vi "PAT Device Software 1.3.vi"() -> ()   [LabVIEW 2018]
uses:
  <vilib>/Utility/error.llb/DialogType.ctl
  <vilib>/DAQmx/write.llb/DAQmx Write (Analog 1D DBL NChan 1Samp).vi
  <vilib>/DAQmx/read.llb/DAQmx Read (Analog 1D DBL NChan 1Samp).vi
  <vilib>/DAQmx/write.llb/DAQmx Write (Analog DBL 1Chan 1Samp).vi
  <vilib>/Analysis/baseanly.llb/Mean (DBL).vi
  <vilib>/Instr/_visa.llb/VISA Configure Serial Port (Instr).vi
  <vilib>/DAQmx/create/channels.llb/DAQmx Create Channel (AO-Voltage-Basic).vi
  <vilib>/DAQmx/create/channels.llb/DAQmx Create Channel (AI-Voltage-Basic).vi
  <vilib>/DAQmx/configure/timing.llb/DAQmx Timing (Sample Clock).vi
  <vilib>/DAQmx/miscellaneous.llb/DAQmx Fill In Error Info.vi
  <vilib>/Analysis/NI_AALBase.lvlib
panel:
  out "CV2 Voltage":dbl format="%#_13g"
  out "CV1 Voltage":dbl format="%#_13g"
  in  "In Progress":bool
  out "Total Test Time":i32
  in  "Test Buffer Duration":i32=10
  in  "Motor Control":bool
  out "Corrected Voltage":dbl=3.0 format="%#_13g"
  out "Rotation Time":dbl format="%#_3g"
  out "Error Ratio":dbl format="%#_13g"
  out "Reference Voltage":dbl=3.001413381851861 format="%0.2f"
  in  "Target Rotation Time":dbl=2.8 format="%#_13g"
  out "Hit Recorded":bool
  in  "CV2 Output":tag="Dev1/ao0"
  in  "CV1 Output":tag="Dev1/ao1"
  in  "Motor Output":tag="Dev2/ao0"
  in  "Hall Sensor Channel":tag="Dev2/ai3"
  in  "O2 Channel":tag="Dev2/ai2"
  in  "P2 Channel":tag="Dev2/ai1"
  in  "PA Channel":tag="Dev2/ai0"
  in  "Relay Port":refnum<visa-resource-name>="COM9"
  in  "Reset To Default":bool
  in  "Sample Rate":i32=10
  in  "CV2 Channel":tag="Dev1/ai0"
  in  "CV1 Channel":tag="Dev1/ai1"
  in  "TA Channel":tag="Dev1/ai6"
  in  "RHA Channel":tag="Dev1/ai7"
  in  "P1 Channel":tag="Dev1/ai5"
  out "Stop Test":bool=TRUE
  out "Is PAT Test?":bool
  in  "Test Begin":bool
  out "Test Duration":i32
  out "Current Test":string
  out "Test Underway":i32
  out "Number of tests":i32=4
  out "Test List":i16[](array[numeric])=[1, 1, 1, 1, 0, 0]
  out "error out 3":errorcluster
  in  "error in 2":errorcluster
  out "error out 2":errorcluster
  in  "error in":errorcluster
  out "error out":errorcluster
  in  "error in (no error)":errorcluster
  in  "Tab Control":enum32{"PAT Test", "Manual Control"}(tab)
  out "PAT Test Readings":T1 {"B40 S" scale=0.0..100.0; "B15 S" scale=0.0..100.0; "Ex70 S" scale=0.0..100.0; "Ex30 S" scale=0.0..100.0; "In70 S" scale=0.0..100.0; "In30 S" scale=0.0..100.0}
  out "Status":string="Status"
  out "Time":string="Time (s)"
  out "Limit":string="Limit"
  out "Comp":string="Comp"
  out "Units":string="Units"
  out "Measured":string="Measured"
  out "Test Name":string="Test Name"
  out "String 22":string="-0.8"
  out "String 24":string="0.8"
  out "String 23":string="-2.0"
  out "String 26":string="26"
  out "String 25":string="2.0"
  out "String 27":string="89"
  out "String 15":string=">="
  out "String 17":string="<="
  out "String 16":string=">="
  out "String 19":string=">="
  out "String 18":string="<="
  out "String 20":string=">="
  out "String 8":string="in H2O"
  out "String 10":string="in H2O"
  out "String 9":string="in H2O"
  out "String 12":string="% O2"
  out "String 11":string="in H2O"
  out "String 13":string="% O2"
  out "String":string="Inhalation (30lpm)"
  out "String 3":string="Exhalation (30lpm)"
  out "String 2":string="Inhalation (70lpm)"
  out "String 5":string="Breathing (15kft)"
  out "String 4":string="Exhalation (70lpm)"
  out "String 6":string="Breathing (40kft)"
  in  "Start PAT Test":bool
  in  "Stop PAT Test":bool
  out "Test Status:":string
  in  "Results File Location:":path=path "X:/Working/Finn Sowerbutts/Aerox/PAT/CDR Files/PAT Device Software/Test Reports"
  in  "PAT Test Settings":T2={"Test Date:"="24 Jan 2019", "Test Time:"="11:23:54", "Pull Test Date:"="", "Operator:"="", "Production Order No.:"="", "Production Lot:"="", "No. Masks in Lot:"="", "Comments:"="", "Array"=[TRUE, TRUE, TRUE, TRUE, FALSE, FALSE], "Test Parameters:"=enum."Quick Test", "Facepiece Leakage"=0.0}
  in  "Preset Directory:":path=path "X:/Working/Finn Sowerbutts/Aerox/PAT/CDR Files/PAT Device Software/Presets"
  in  "MC Fields":T3={"Test Date:"="24 Jan 2019", "Test Time:"="11:23:54", "Operator:"="", "PAX Serial No.:"="", "Production Lot:"="", "No. Masks in Lot:"="", "Test Duration"=0, "Presets in Directory:"=0, "MC Test Length"=enum."Run Continuously", "Current Preset:"="Breathing Test 2.ini", "Preset Save"=FALSE}
  in  "MC Instrumentation":T4 {"Motor Speed:" min=0.0 max=3.0 step=0.25; "F2 Leakage" min=0.0 max=150.0 step=1.0; "CV2 Flow Rate:" min=0.0 max=100.0 step=10.0; "CV1 Flow Rate:" min=0.0 max=5.0 step=0.5}
  in  "Start Custom Test":bool
  in  "Stop Custom Test":bool
  # "ccm"
  # "s"
  # "Pamb"
  # "Tamb"
  # "Hamb"
  # "in H2O"
  # "°C"
  # "%"
  # "F2"
  # "ccm"
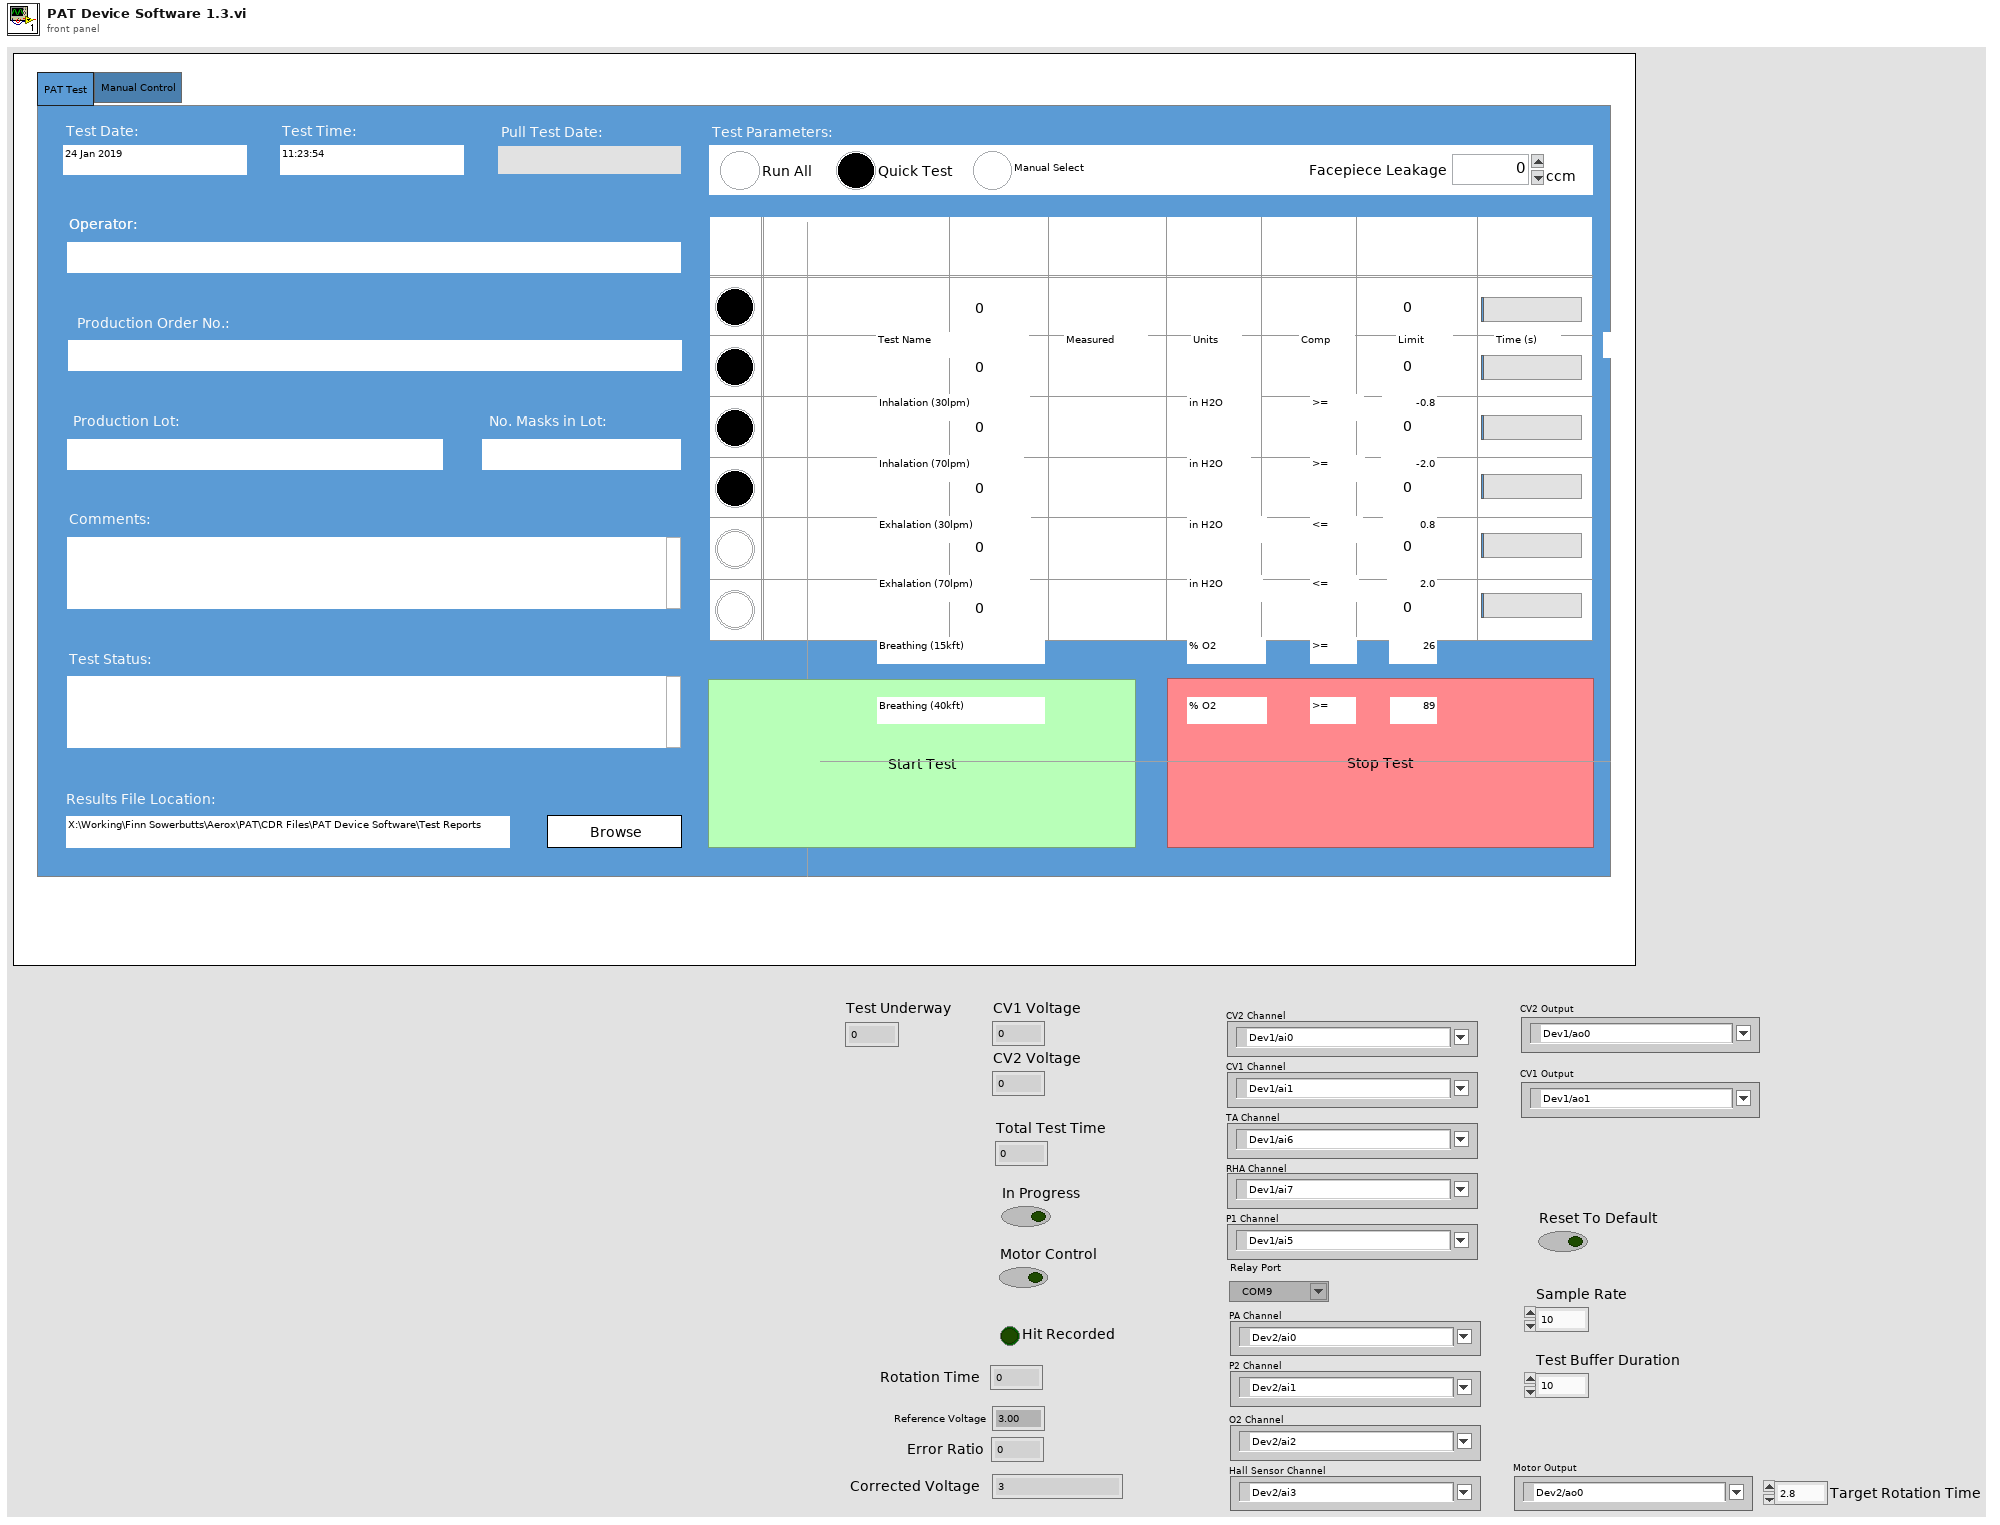
[diagram p1: front panel]
types:
  T1 = cluster{"In30 M":dbl, "In30 T":i64, "In30 S":u8, "In70 M":dbl, "Ex30 M":dbl, "Ex70 M":dbl, "B40 M":dbl, "B15 M":dbl, "In70 T":i64, "Ex30 T":i64, "Ex70 T":i64, "B40 T":i64, "B15 T":i64, "In70 S":u8, "Ex30 S":u8, "Ex70 S":u8, "B15 S":u8, "B40 S":u8}
  T2 = cluster{"Test Date:":string, "Test Time:":string, "Pull Test Date:":string, "Operator:":string, "Production Order No.:":string, "Production Lot:":string, "No. Masks in Lot:":string, "Comments:":string, "Array":bool[], "Test Parameters:":enum32{"Run All", "Quick Test", "Manual Select"}, "Facepiece Leakage":dbl}
  T3 = cluster{"Test Date:":string, "Test Time:":string, "Operator:":string, "PAX Serial No.:":string, "Production Lot:":string, "No. Masks in Lot:":string, "Test Duration":i64, "Presets in Directory:":i32, "MC Test Length":enum32{"Run Continuously", "Run for:"}, "Current Preset:":string, "Preset Save":bool}
  T4 = cluster{"SV1":bool, "SV2":bool, "SV3":bool, "SV4":bool, "SV5":bool, "SV6":bool, "SV7":bool, "SV8":bool, "SV9":bool, "M1":bool, "MP1":bool, "MP2":bool, "CV1":bool, "CV2":bool, "CV1 Flow Rate:":dbl, "CV2 Flow Rate:":dbl, "P2 Pressure:":dbl, "O2 Concentration:":dbl, "Ambient Pressure:":dbl, "Ambient Temp.:":dbl, "Ambient Humidity:":dbl, "Motor Speed:":dbl, "F2 Leakage":dbl, "P1 Pressure:":dbl}
  T5 = enum8{"Enabled", "Disabled", "Disabled and Grayed Out"}
  T6 = typedef "DialogType.ctl" = u16
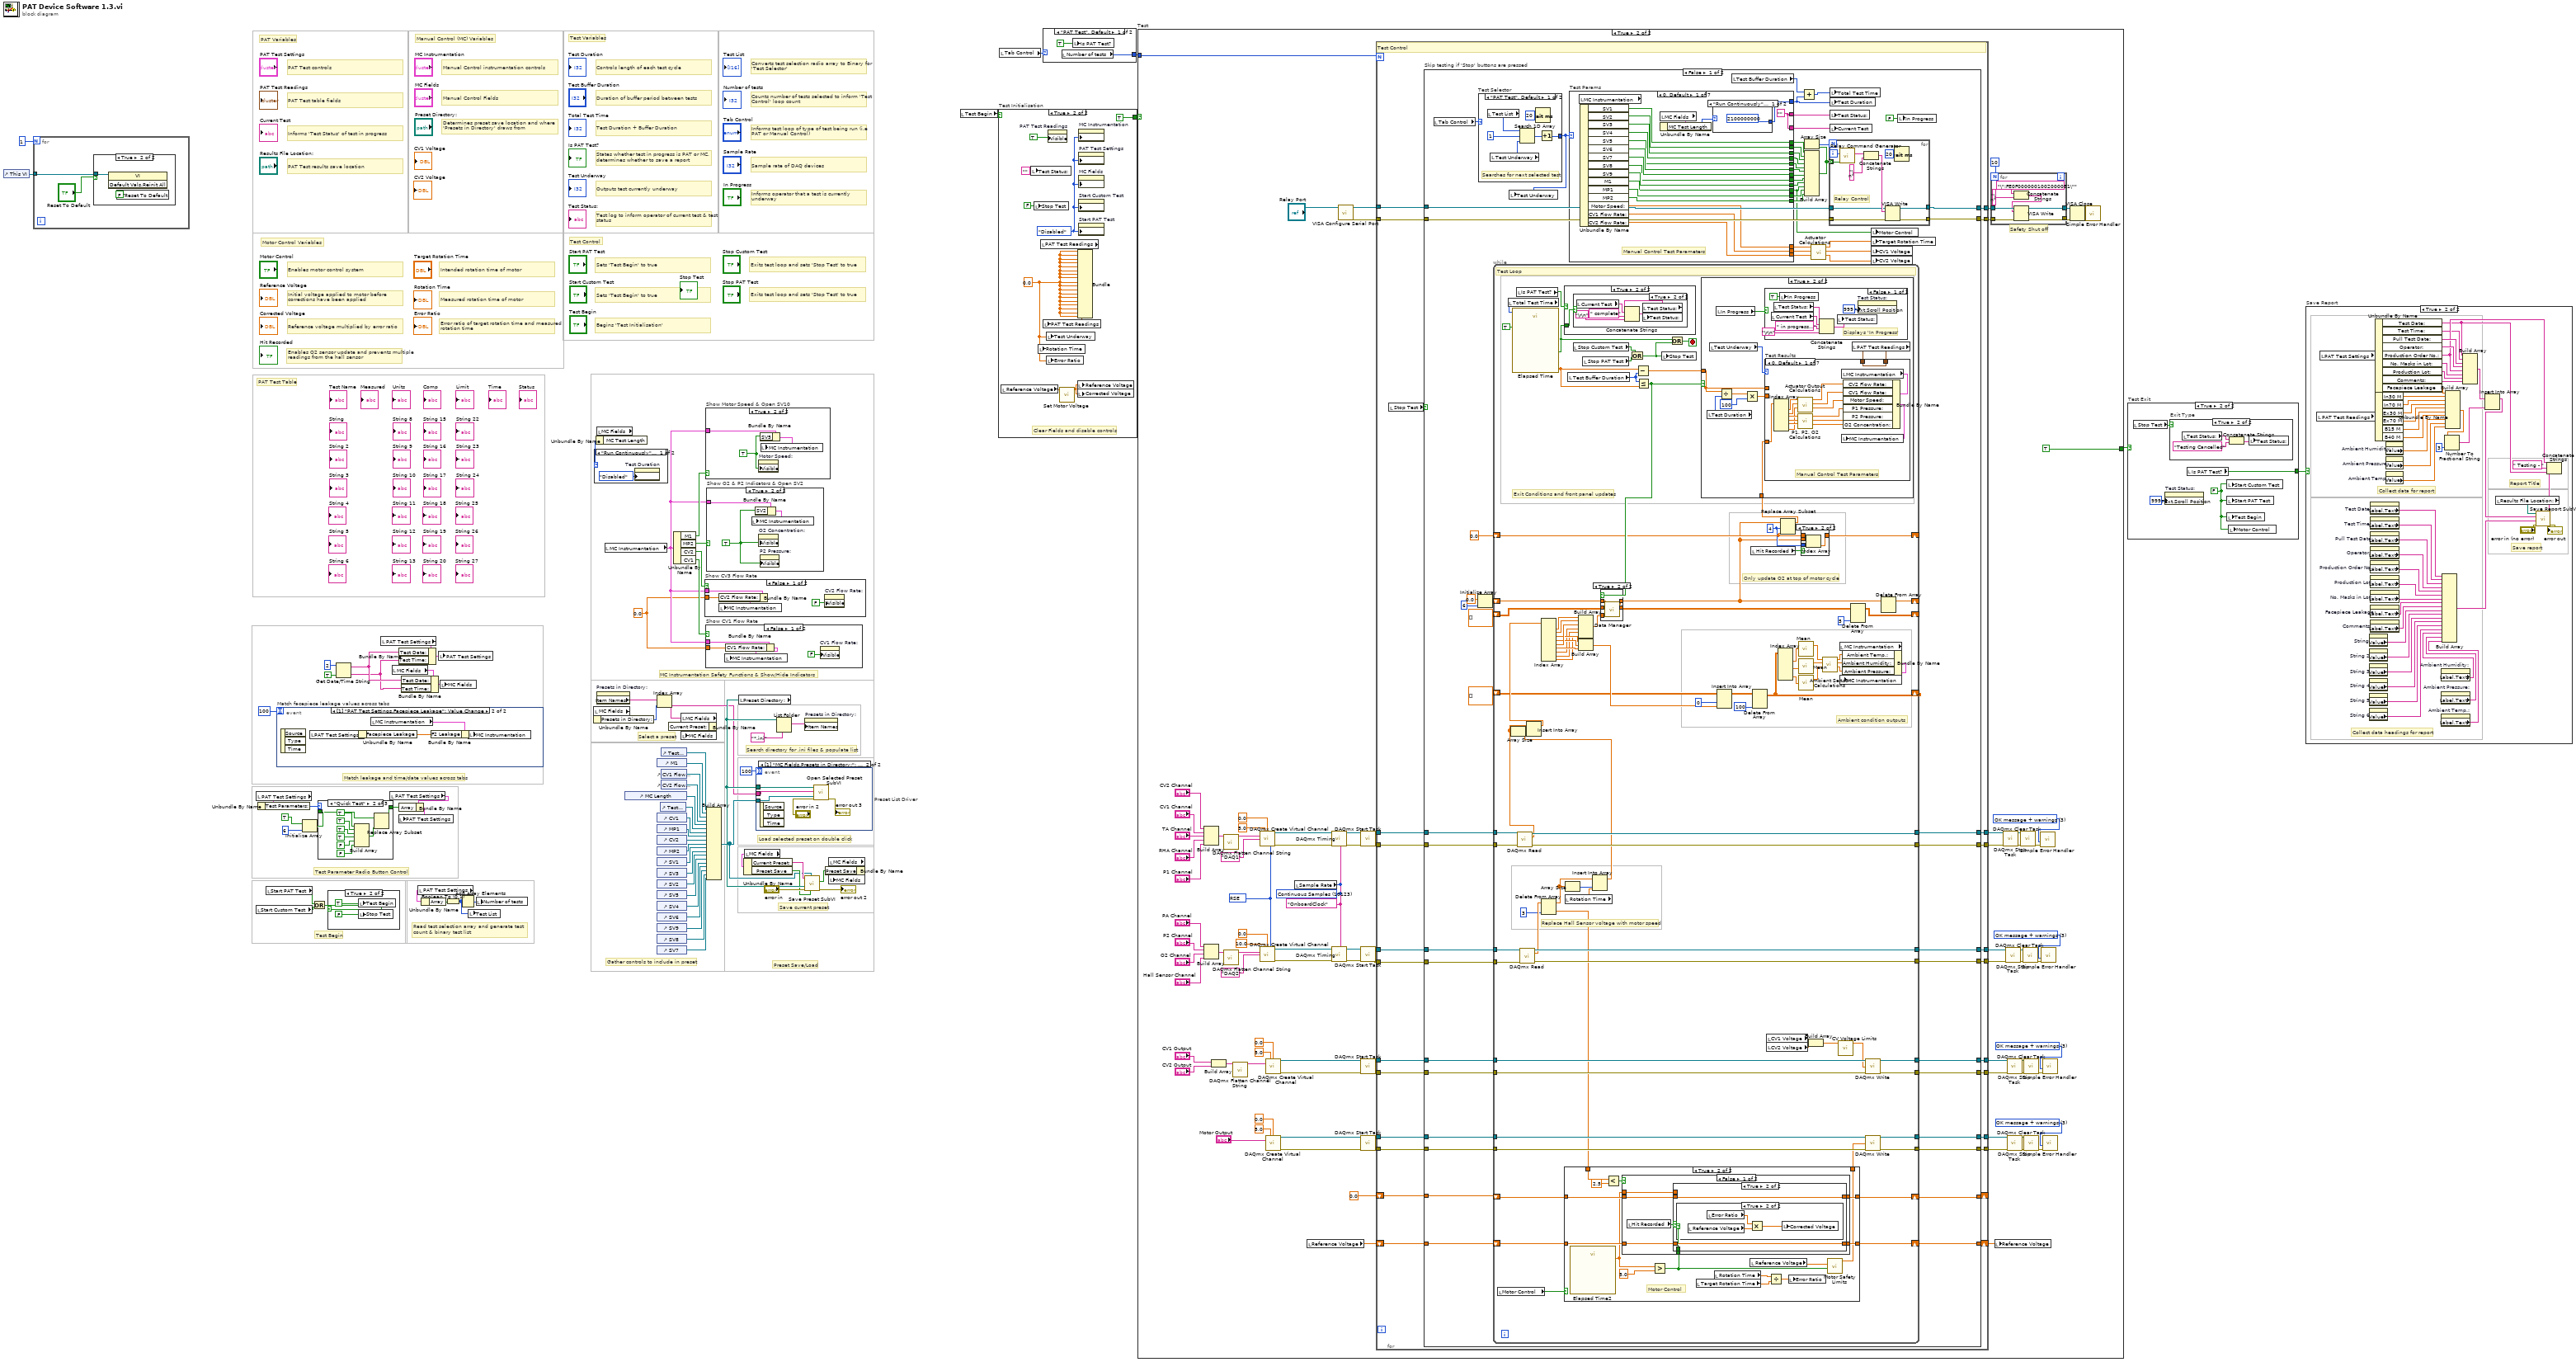
[diagram p0: block diagram]
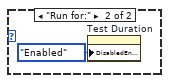
[diagram p2: hidden frame]
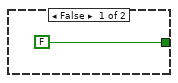
[diagram p4: hidden frame]
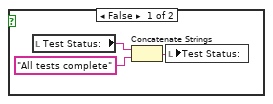
[diagram p5: hidden frame]
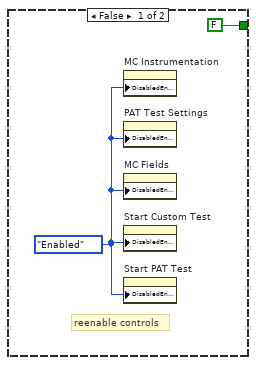
[diagram p6: hidden frame]
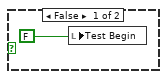
[diagram p7: hidden frame]
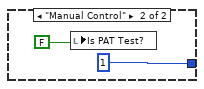
[diagram p8: hidden frame]
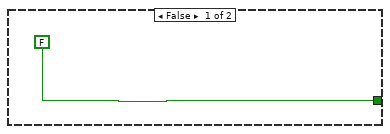
[diagram p9: hidden frame]
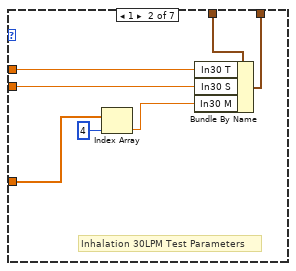
[diagram p14: hidden frame]
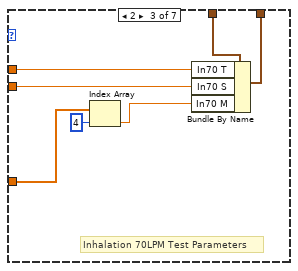
[diagram p15: hidden frame]
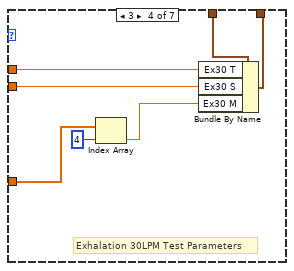
[diagram p16: hidden frame]
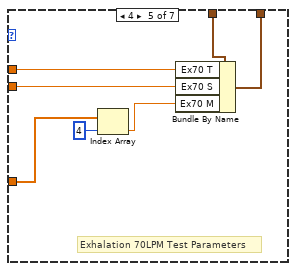
[diagram p17: hidden frame]
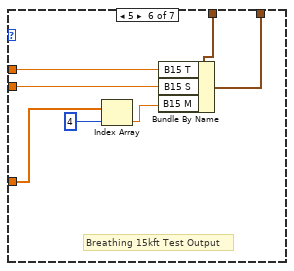
[diagram p18: hidden frame]
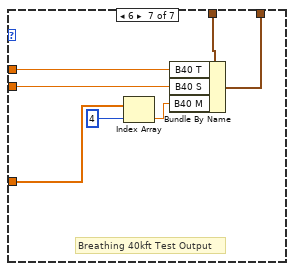
[diagram p19: hidden frame]
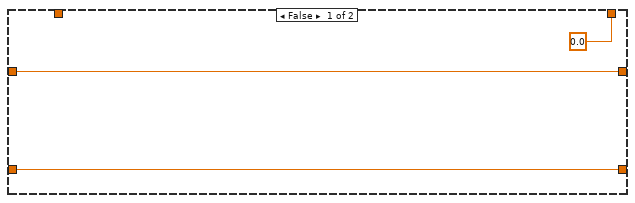
[diagram p20: hidden frame]
diagram:
  w1 = 0.0
  # "Enables O2 sensor update and prevents multiple readings from the hall sensor"
  # "Error ratio of target rotation time and measured rotation time"
  # "Measured rotation time of motor"
  # "Intended rotation time of motor"
  # "Reference voltage multiplied by error ratio"
  # "Initial voltage applied to motor before corrections have been applied"
  # "Enables motor control system"
  # "Motor Control Variables"
  # "Informs operator that a test is currently underway"
  # "Sample rate of DAQ devices"
  # "Test log to inform operator of current test & test status"
  # "Outputs test currently underway"
  # "Test Duration + Buffer Duration"
  # "Duration of buffer period between tests"
  # "Preset Save/Load"
  # "Save current preset"
  # "Load selected preset on double click"
  # "Search directory for .ini files & populate list"
  # "Gather controls to include in preset"
  # "Select a preset"
  # "Read test selection array and generate test count & binary test list"
  # "MC Instrumentation Safety Functions & Show/Hide Indicators"
  # "Determines preset save location and where 'Presets in Directory' draws from"
  # "Test Control"
  # "Exits test loop and sets 'Stop Test' to true"
  # "Exits test loop and sets 'Stop Test' to true"
  # "Sets 'Test Begin' to true"
  # "Sets 'Test Begin' to true"
  # "PAT Test results save location"
  # "Informs test loop of type of test being run (i.e PAT or Manual Control)"
  # "Counts number of tests selected to inform 'Test Control' loop count"
  # "Begins 'Test Initialisation'"
  # "States whether test in progress is PAT or MC, determines whether to save a report"
  # "Controls length of each test cycle"
  # "Converts test selection radio array to Binary for 'Test Selector'"
  # "Test Begin"
  # "Test Variables"
  # "Manual Control Fields"
  # "Manual Control instrumentation controls"
  # "PAT Test controls"
  # "PAT Test table fields"
  # "Informs 'Test Status' of test in progress"
  # "Manual Control (MC) Variables"
  # "Test Parameter Radio Button Control"
  # "Match leakage and time/date values across tabs"
  # "PAT Variables"
  # "PAT Test Table"
  n1 = control-ref of="This VI"() -> (w18:refnum<vi>)
  n2 = for {
    N: 1 -> [_]
    tunnel: w18 -> [w80]
    n3 = case shown="True" "Reset To Default" {
      tunnel: w80 -> [_ w82]
      frame False {
      }
      frame True {
        n4 = invoke class="VI" method="Default Vals.Reinit All"(reference=w82) -> ()  [unwired: 2 in, 3 out]
        n5 = local write "Reset To Default"(FALSE ("Boolean")) -> ()
      }
    }
  }
  n6 = local read "Start Custom Test"() -> (w27:bool)
  n7 = local read "PAT Test Settings"() -> (w50:T2)
  n8 = Unbundle By Name(w50) -> ("Test Parameters:"=w46:enum32{"Run All", "Quick Test", "Manual Select"})
  n9 = local read "Start PAT Test"() -> (w28:bool)
  n10 = event "Match facepiece leakage values across tabs" shown="[1] \"PAT Test Settings.Facepiece Leakage\": Value Change" {
    selector: _ -> [_ _]
    dyn-events: _ -> [_ _]
    timeout: 100 -> [_ _]
    event Timeout {
      n11 = event-data() -> ()  [unwired: 1 in, 3 out]
    }
    event "PAT Test Settings.Facepiece Leakage": Value Change {
      n12 = event-data() -> ()  [unwired: 1 in, 3 out]
      n13 = local read "PAT Test Settings"() -> (w84:T2)
      n14 = Unbundle By Name(w84) -> ("Facepiece Leakage"=w83:dbl)
      n15 = local read "MC Instrumentation"() -> (w85:T4)
      n16 = Bundle By Name(cluster=w85, "F2 Leakage"=w83) -> (w86:T4)
      n17 = local write "MC Instrumentation"(w86) -> ()
    }
  }
  n18 = Initialize Array(TRUE, 6) -> (w76:bool[])
  n19 = Or(x=w28, y=w27) -> (x .or. y?=w33:bool)
  n20 = case shown="\"Quick Test\"" w46 {
    tunnel: [w87 w90 w99] -> w47
    tunnel: w76 -> [w87 w88 w100]
    frame "Run All", Default {
    }
    frame "Quick Test" {
      n21 = Build Array(TRUE, TRUE, TRUE, TRUE, FALSE, FALSE) -> (w89:bool[])
      n22 = Replace Array Subset(array=w88, new element=w89) -> (w90:bool[])  [unwired: 1 in]
    }
    frame "Manual Select" {
      n23 = local read "PAT Test Settings"() -> (w98:T2)
      n24 = Unbundle By Name(w98) -> ("Array"=w97:bool[])
      n25 = Replace Array Subset(array=w100, new element=w97) -> (w99:bool[])  [unwired: 1 in]
    }
  }
  n26 = case shown="True" w33 {
    frame False {
      n27 = local write "Test Begin"(FALSE) -> ()
    }
    frame True {
      n28 = local write "Test Begin"(TRUE) -> ()
      n29 = local write "Stop Test"(FALSE) -> ()
    }
  }
  n30 = Get Date/Time String(date format (0)=2, want seconds? (F)=TRUE) -> (date string=w35:string, time string=w34:string)  [unwired: 1 in]
  n31 = local read "PAT Test Settings"() -> (w52:T2)
  n32 = local read "PAT Test Settings"() -> (w49:T2)
  n33 = local read "MC Fields"() -> (w41:T3)
  n34 = Bundle By Name(cluster=w52, "Test Date:"=w35, "Test Time:"=w34) -> (w51:T2)
  n35 = Bundle By Name(cluster=w49, "Array"=w47) -> (w48:T2)
  n36 = local write "PAT Test Settings"(w48) -> ()
  n37 = Bundle By Name(cluster=w41, "Test Date:"=w35, "Test Time:"=w34) -> (w40:T3)
  n38 = local read "PAT Test Settings"() -> (w32:T2)
  n39 = Unbundle By Name(w32) -> ("Array"=w43:bool[])
  n40 = local write "PAT Test Settings"(w51) -> ()
  n41 = local write "MC Fields"(w40) -> ()
  n42 = Boolean To (0,1)(Boolean=w43) -> (0, 1=w30:i16[])
  n43 = Add Array Elements(numeric array=w30) -> (sum=w31:i16)
  n44 = local write "Test List"(w30) -> ()
  n45 = local write "Number of tests"(w31) -> ()
  n46 = local read "MC Fields"() -> (w37:T3)
  n47 = Unbundle By Name(w37) -> ("Presets in Directory:"=w36:i32)
  n48 = local read "MC Fields"() -> (w8:T3)
  n49 = Unbundle By Name(w8) -> ("MC Test Length"=w7:enum32{"Run Continuously", "Run for:"})
  n50 = case shown="\"Run Continuously\", Default" w7 {
    frame "Run Continuously", Default {
      n51 = property on="Test Duration" class="DigNum (strict)"("DisabledEnum"=T5."Disabled" ("Disabled")) -> ()  [unwired: 2 in, 2 out]
    }
    frame "Run for:" {
      n52 = property on="Test Duration" class="DigNum (strict)"("DisabledEnum"=T5."Enabled" ("Disabled")) -> ()  [unwired: 2 in, 2 out]
    }
  }
  n53 = property on="Presets in Directory:" class="LstBox (strict)"() -> ("Item Names"=w56:string[])  [unwired: 2 in, 2 out]
  n54 = local read "MC Instrumentation"() -> (w2:T4)
  n55 = control-ref of="MC Length"() -> (w39:refnum<vi>)
  n56 = Index Array(array=w56, index=w36) -> (element=w17:string)
  n57 = control-ref of="M1"() -> (w72:refnum<vi>)
  n58 = control-ref of="CV1"() -> (w6:refnum<vi>)
  n59 = control-ref of="MP1"() -> (w68:refnum<vi>)
  n60 = control-ref of="CV2"() -> (w69:refnum<vi>)
  n61 = control-ref of="MP2"() -> (w67:refnum<vi>)
  n62 = control-ref of="SV1"() -> (w66:refnum<vi>)
  n63 = control-ref of="SV3"() -> (w65:refnum<vi>)
  n64 = control-ref of="SV2"() -> (w64:refnum<vi>)
  n65 = control-ref of="SV5"() -> (w63:refnum<vi>)
  n66 = control-ref of="SV4"() -> (w62:refnum<vi>)
  n67 = control-ref of="SV6"() -> (w61:refnum<vi>)
  n68 = control-ref of="SV9"() -> (w60:refnum<vi>)
  n69 = control-ref of="SV8"() -> (w59:refnum<vi>)
  n70 = control-ref of="SV7"() -> (w58:refnum<vi>)
  n71 = control-ref of="Test Duration"() -> (w38:refnum<vi>)
  n72 = control-ref of="Test Duration"() -> (w73:refnum<vi>)
  n73 = control-ref of="CV1 Flow Rate:"() -> (w71:refnum<vi>)
  n74 = control-ref of="CV2 Flow Rate:"() -> (w70:refnum<vi>)
  n75 = Unbundle By Name(w2) -> ("M1"=w44:bool, "MP2"=w4:bool, "CV2"=w3:bool, "CV1"=w45:bool)
  n76 = local read "MC Fields"() -> (w16:T3)
  n77 = Bundle By Name(cluster=w16, "Current Preset:"=w17) -> (w15:T3)
  n78 = local write "MC Fields"(w15) -> ()
  n79 = case "Show CV3 Flow Rate" shown="False" w3 {
    tunnel: w2 -> [w108 _]
    tunnel: w1 -> [w106 _]
    frame False {
      n80 = Bundle By Name(cluster=w108, "CV2 Flow Rate:"=w106) -> (w109:T4)
      n81 = local write "MC Instrumentation"(w109) -> ()
      n82 = property on="CV2 Flow Rate:" class="DigNum (strict)"("Visible"=FALSE) -> ()  [unwired: 2 in, 2 out]
    }
    frame True {
      n83 = property on="CV2 Flow Rate:" class="DigNum (strict)"("Visible"=TRUE) -> ()  [unwired: 2 in, 2 out]
    }
  }
  n84 = case "Show Motor Speed & Open SV10" shown="True" w44 {
    tunnel: w2 -> [_ w112]
    frame False {
      n85 = property on="Motor Speed:" class="DigNum (strict)"("Visible"=FALSE) -> ()  [unwired: 2 in, 2 out]
    }
    frame True {
      w113 = TRUE ("Visible")
      n86 = property on="Motor Speed:" class="DigNum (strict)"("Visible"=w113) -> ()  [unwired: 2 in, 2 out]
      n87 = Bundle By Name(cluster=w112, "SV5"=w113) -> (w114:T4)
      n88 = local write "MC Instrumentation"(w114) -> ()
    }
  }
  n89 = case "Show CV1 Flow Rate" shown="False" w45 {
    tunnel: w2 -> [w117 _]
    tunnel: w1 -> [w115 _]
    frame False {
      n90 = Bundle By Name(cluster=w117, "CV1 Flow Rate:"=w115) -> (w116:T4)
      n91 = local write "MC Instrumentation"(w116) -> ()
      n92 = property on="CV1 Flow Rate:" class="DigNum (strict)"("Visible"=FALSE) -> ()  [unwired: 2 in, 2 out]
    }
    frame True {
      n93 = property on="CV1 Flow Rate:" class="DigNum (strict)"("Visible"=TRUE) -> ()  [unwired: 2 in, 2 out]
    }
  }
  n94 = Build Array(w73, w72, w71, w70, w39, w38, w6, w68, w69, w67, w66, w65, w64, w63, w62, w61, w60, w59, w58) -> (w5:refnum<vi>[])
  n95 = case "Show O2 & P2 Indicators & Open SV2" shown="True" w4 {
    tunnel: w2 -> [_ w121]
    frame False {
      w120 = FALSE ("Visible")
      n96 = property on="O2 Concentration:" class="DigNum (strict)"("Visible"=w120) -> ()  [unwired: 2 in, 2 out]
      n97 = property on="P2 Pressure:" class="DigNum (strict)"("Visible"=w120) -> ()  [unwired: 2 in, 2 out]
    }
    frame True {
      w122 = TRUE ("Visible")
      n98 = Bundle By Name(cluster=w121, "SV2"=w122) -> (w123:T4)
      n99 = local write "MC Instrumentation"(w123) -> ()
      n100 = property on="O2 Concentration:" class="DigNum (strict)"("Visible"=w122) -> ()  [unwired: 2 in, 2 out]
      n101 = property on="P2 Pressure:" class="DigNum (strict)"("Visible"=w122) -> ()  [unwired: 2 in, 2 out]
    }
  }
  n102 = local read "Preset Directory:"() -> (w21:path)
  n103 = local read "MC Fields"() -> (w14:T3)
  n104 = Unbundle By Name(w14) -> ("Current Preset:"=w13:string, "Preset Save"=w12:bool)
  n105 = event "Preset List Driver" shown="[1] \"MC Fields.Presets in Directory:\": Double Click" {
    selector: _ -> [_ _]
    dyn-events: _ -> [_ _]
    timeout: 100 -> [_ _]
    tunnel: w17 -> [_ w126]
    tunnel: w21 -> [_ w127]
    tunnel: w5 -> [_ w124]
    event Timeout {
      n106 = event-data() -> ()  [unwired: 1 in, 3 out]
    }
    event "MC Fields.Presets in Directory:": Double Click {
      n107 = event-data() -> ()  [unwired: 1 in, 3 out]
      n108 = call "Open Selected Preset SubVI.vi"("error in (no error)"="error in 2", "Controls"=w124, "Current Preset"=w126, "Preset Directory:"=w127) -> ("error out"=→"error out 3":errorcluster)  [unwired: 7 in]
    }
  }
  n109 = List Folder(path=w21, pattern="*.ini") -> (filenames=w55:string[])  [unwired: 2 in, 3 out]
  n110 = property on="Presets in Directory:" class="LstBox (strict)"("Item Names"=w55) -> ()  [unwired: 2 in, 2 out]
  n111 = call "Save Preset SubVI.vi"("Preset Save"=w12, "Control Settings"=w5, "error in (no error)"="error in", "Preset Directory:"=w21, "Preset Name"=w13) -> ("error out"=→"error out 2":errorcluster, "Reset 'Preset Save'"=w9:bool)  [unwired: 5 in]
  n112 = local read "MC Fields"() -> (w10:T3)
  n113 = Bundle By Name(cluster=w10, "Preset Save"=w9) -> (w11:T3)
  n114 = local write "MC Fields"(w11) -> ()
  n115 = local read "Test Begin"() -> (w26:bool)
  n116 = case "Test Initialisation" shown="True" w26 {
    tunnel: [FALSE TRUE] -> w24
    frame False {
      w129 = T5."Enabled" ("Disabled")
      # "reenable controls"
      n117 = property on="MC Instrumentation" class="Clust (strict)"("DisabledEnum"=w129) -> ()  [unwired: 2 in, 2 out]
      n118 = property on="PAT Test Settings" class="Clust (strict)"("DisabledEnum"=w129) -> ()  [unwired: 2 in, 2 out]
      n119 = property on="MC Fields" class="Clust (strict)"("DisabledEnum"=w129) -> ()  [unwired: 2 in, 2 out]
      n120 = property on="Start Custom Test" class="Bool (strict)"("DisabledEnum"=w129) -> ()  [unwired: 2 in, 2 out]
      n121 = property on="Start PAT Test" class="Bool (strict)"("DisabledEnum"=w129) -> ()  [unwired: 2 in, 2 out]
    }
    frame True {
      w133 = 0.0
      w135 = T5."Disabled" ("Disabled")
      # "Clear Fields and disable controls"
      n122 = local read "Reference Voltage"() -> (w131:dbl)
      n123 = local write "Test Status:"("") -> ()
      n124 = local write "Stop Test"(FALSE ("Visible")) -> ()
      n125 = local write "Rotation Time"(w133) -> ()
      n126 = local read "PAT Test Readings"() -> (w140:T1)
      n127 = local write "Test Underway"(w133) -> ()
      n128 = local write "Error Ratio"(w133) -> ()
      n129 = property on="PAT Test Readings" class="Clust (strict)"("Visible"=TRUE) -> ()  [unwired: 2 in, 2 out]
      n130 = call "Set Motor Voltage.vi"("Reference Voltage in"=w131) -> ("Reference Voltage out"=w132:dbl)  [unwired: 10 in]
      n131 = local write "Reference Voltage"(w132) -> ()
      n132 = local write "Corrected Voltage"(w132) -> ()
      n133 = Bundle(cluster=w140, "In30 M"=w133, "In30 T"=w133, "In30 S"=w133, "In70 M"=w133, "Ex30 M"=w133, "Ex70 M"=w133, "B40 M"=w133, "B15 M"=w133, "In70 T"=w133, "Ex30 T"=w133, "Ex70 T"=w133, "B40 T"=w133, "B15 T"=w133, "In70 S"=w133, "Ex30 S"=w133, "Ex70 S"=w133, "B15 S"=w133, "B40 S"=w133) -> (w139:T1)
      n134 = local write "PAT Test Readings"(w139) -> ()
      n135 = property on="MC Instrumentation" class="Clust (strict)"("DisabledEnum"=w135) -> ()  [unwired: 2 in, 2 out]
      n136 = property on="PAT Test Settings" class="Clust (strict)"("DisabledEnum"=w135) -> ()  [unwired: 2 in, 2 out]
      n137 = property on="MC Fields" class="Clust (strict)"("DisabledEnum"=w135) -> ()  [unwired: 2 in, 2 out]
      n138 = property on="Start Custom Test" class="Bool (strict)"("DisabledEnum"=w135) -> ()  [unwired: 2 in, 2 out]
      n139 = property on="Start PAT Test" class="Bool (strict)"("DisabledEnum"=w135) -> ()  [unwired: 2 in, 2 out]
    }
  }
  n140 = local read "Tab Control"() -> (w29:enum32{"PAT Test", "Manual Control"})
  n141 = case shown="\"PAT Test\", Default" w29 {
    tunnel: [w142 1] -> w42
    frame "PAT Test", Default {
      n142 = local read "Number of tests"() -> (w142:i32)
      n143 = local write "Is PAT Test?"(TRUE ("Boolean")) -> ()
    }
    frame "Manual Control" {
      n144 = local write "Is PAT Test?"(FALSE ("Boolean")) -> ()
    }
  }
  n145 = case "Test" shown="True" w24 {
    tunnel: w42 -> [_ w235]
    tunnel: [FALSE TRUE] -> w25
    frame False {
    }
    frame True {
      w156 = T6 3 items=["no dialog", "OK message", "continue or stop message", "OK message + warnings", "continue/stop + warnings"] ("type of dialog (OK msg:1)")
      w154 = 10083 items=["Default"=-1, "RSE"=10083, "NRSE"=10078, "Differential"=10106, "Pseudodifferential"=12529] ("input terminal configuration")
      w153 = tag "OnboardClock" ("source")
      w196 = T6 3 items=["no dialog", "OK message", "continue or stop message", "OK message + warnings", "continue/stop + warnings"] ("type of dialog (OK msg:1)")
      w197 = T6 3 items=["no dialog", "OK message", "continue or stop message", "OK message + warnings", "continue/stop + warnings"] ("type of dialog (OK msg:1)")
      w199 = T6 3 items=["no dialog", "OK message", "continue or stop message", "OK message + warnings", "continue/stop + warnings"] ("type of dialog (OK msg:1)")
      w151 = 10123 items=["Finite Samples"=10178, "Continuous Samples"=10123, "Hardware Timed Single Point"=12522] ("sample mode")
      # "Safety Shut off"
      n146 = Build Array("CV2 Channel", "CV1 Channel", "TA Channel", "RHA Channel", "P1 Channel") -> (w217:tag[])
      n147 = Build Array("PA Channel", "P2 Channel", "O2 Channel", "Hall Sensor Channel") -> (w168:tag[])
      n148 = Build Array("CV1 Output", "CV2 Output") -> (w188:tag[])
      n149 = call <vilib>:"DAQmx Flatten Channel String.vi"("names in"=w217) -> ("names out"=w218:string)  [unwired: 13 in, 1 out]
      n150 = call <vilib>:"DAQmx Flatten Channel String.vi"("names in"=w168) -> ("names out"=w176:string)  [unwired: 13 in, 1 out]
      n151 = call <vilib>:"DAQmx Flatten Channel String.vi"("names in"=w188) -> ("names out"=w181:string)  [unwired: 13 in, 1 out]
      n152 = call-poly <vilib>:"DAQmx Create Virtual Channel.vi"("maximum value"=5.0, "minimum value"=0.0, "input terminal configuration"=w154, "physical channels"=w218, "name to assign"="DAQ1") -> ("task out"=w232:refnum<k21>, "error out"=w233:errorcluster)  [unwired: 9 in]
      n153 = call-poly <vilib>:"DAQmx Create Virtual Channel.vi"("maximum value"=10.0, "minimum value"=0.0, "input terminal configuration"=w154, "physical channels"=w176, "name to assign"="DAQ2") -> ("task out"=w175:refnum<k21>, "error out"=w174:errorcluster)  [unwired: 9 in]
      n154 = call-poly <vilib>:"DAQmx Create Virtual Channel.vi"("maximum value"=5.0, "minimum value"=0.0, "physical channels"=w181) -> ("task out"=w191:refnum<k21>, "error out"=w192:errorcluster)  [unwired: 11 in]
      n155 = call-poly <vilib>:"DAQmx Create Virtual Channel.vi"("maximum value"=5.0, "minimum value"=0.0, "physical channels"="Motor Output") -> ("task out"=w161:refnum<k21>, "error out"=w160:errorcluster)  [unwired: 11 in]
      n156 = local read "Sample Rate"() -> (w152:i32)
      n157 = local read "Reference Voltage"() -> (w147:dbl)
      n158 = call-poly <vilib>:"DAQmx Timing.vi"("task/channels in"=w232, "sample mode"=w151, "rate"=w152, "source"=w153, "error in"=w233) -> ("task out"=w180:refnum<k21>, "error out"=w179:errorcluster)  [unwired: 9 in]
      n159 = call-poly <vilib>:"DAQmx Timing.vi"("task/channels in"=w175, "sample mode"=w151, "rate"=w152, "source"=w153, "error in"=w174) -> ("task out"=w177:refnum<k21>, "error out"=w178:errorcluster)  [unwired: 9 in]
      n160 = call-poly "VISA Configure Serial Port"("VISA resource name"="Relay Port") -> ("VISA resource name out"=w214:refnum<visa-resource-name>, "error out"=w213:errorcluster)  [unwired: 13 in]
      n161 = call <vilib>:"DAQmx Start Task.vi"("task/channels in"=w180, "error in"=w179) -> ("task out"=w224:refnum<k21>, "error out"=w225:errorcluster)  [unwired: 12 in]
      n162 = call <vilib>:"DAQmx Start Task.vi"("task/channels in"=w177, "error in"=w178) -> ("task out"=w170:refnum<k21>, "error out"=w169:errorcluster)  [unwired: 12 in]
      n163 = call <vilib>:"DAQmx Start Task.vi"("task/channels in"=w191, "error in"=w192) -> ("task out"=w185:refnum<k21>, "error out"=w184:errorcluster)  [unwired: 12 in]
      n164 = call <vilib>:"DAQmx Start Task.vi"("task/channels in"=w161, "error in"=w160) -> ("task out"=w164:refnum<k21>, "error out"=w165:errorcluster)  [unwired: 12 in]
      n165 = for {
        N: w235 -> [_]
        tunnel: w224 -> [w266]
        tunnel: w225 -> [w265]
        tunnel: [w264] -> w229
        tunnel: [w263] -> w228
        tunnel: w214 -> [w262]
        tunnel: w213 -> [w261]
        tunnel: [w259] -> w210
        tunnel: [w260] -> w209
        tunnel: [w258] -> w204
        tunnel: [w257] -> w203
        tunnel: w170 -> [w256]
        tunnel: w169 -> [w255]
        tunnel: w185 -> [w254]
        tunnel: w184 -> [w253]
        tunnel: [w252] -> w183
        tunnel: [w251] -> w182
        tunnel: w164 -> [w247]
        tunnel: w165 -> [w248]
        tunnel: [w249] -> w166
        tunnel: [w250] -> w167
        shift-right: [w244] -> _
        shift-left: 0.0 ("element") -> [w246]
        shift-right: [w243] -> w146
        shift-left: w147 -> [w245]
        # "Test Control"
        n166 = local read "Stop Test"() -> (w267:bool)
        n167 = case "Skip testing if 'Stop' buttons are pressed" shown="False" w267 {
          tunnel: w266 -> [w324 w726]
          tunnel: w265 -> [w323 w725]
          tunnel: [w322 w726] -> w264
          tunnel: [w321 w725] -> w263
          tunnel: [w303 w723] -> w259
          tunnel: [w302 w724] -> w260
          tunnel: w262 -> [w301 w724]
          tunnel: w261 -> [w300 w723]
          tunnel: [w299 w722] -> w258
          tunnel: [w298 w721] -> w257
          tunnel: w256 -> [w297 w722]
          tunnel: w255 -> [w296 w721]
          tunnel: w254 -> [w295 w720]
          tunnel: w253 -> [w294 w719]
          tunnel: [w293 w720] -> w252
          tunnel: [w292 w719] -> w251
          tunnel: w247 -> [w288 w718]
          tunnel: w248 -> [w289 w717]
          tunnel: [w290 w718] -> w249
          tunnel: [w291 w717] -> w250
          tunnel: w246 -> [w283 w716]
          tunnel: w245 -> [w282 w715]
          tunnel: [w281 w716] -> w244
          tunnel: [w280 w715] -> w243
          frame False {
            n168 = local read "Tab Control"() -> (w325:enum32{"PAT Test", "Manual Control"})
            n169 = Initialize Array(0.0 ("element"), 6 ("dimension size")) -> (w284:dbl[])
            n170 = case "Test Selector" shown="\"PAT Test\", Default" w325 {
              tunnel: [w709 0] -> w319
              frame "PAT Test", Default {
                # "Searches for next selected test"
                n171 = local read "Test List"() -> (w710:i16[])
                n172 = local read "Test Underway"() -> (w711:i32)
                n173 = Search 1D Array(1D array=w710, element=1, start index (0)=w711) -> (index of element=w713:i32)
                n174 = Wait (ms)(milliseconds to wait=u32 20) -> ()  [unwired: 1 out]
                n175 = Increment(x=w713) -> (x+1=w709:i32)
              }
              frame "Manual Control" {
              }
            }
            n176 = while {
              tunnel: w324 -> [w415]
              tunnel: w323 -> [w414]
              tunnel: [w412] -> w322
              tunnel: [w413] -> w321
              shift-right: [w377] -> _
              shift-left: w284 -> [w410]
              shift-right: [w378] -> _
              shift-left: dbl[][] [] -> [w411]
              shift-right: [w337] -> _
              shift-left: dbl[][] [] -> [w346]
              tunnel: [w395] -> w299
              tunnel: [w394] -> w298
              tunnel: w297 -> [w393]
              tunnel: w296 -> [w392]
              tunnel: w295 -> [w391]
              tunnel: w294 -> [w390]
              tunnel: [w389] -> w293
              tunnel: [w388] -> w292
              tunnel: w288 -> [w382]
              tunnel: w289 -> [w383]
              tunnel: [w384] -> w290
              tunnel: [w385] -> w291
              shift-right: [w372] -> w280
              shift-left: w282 -> [w370]
              shift-right: [w373] -> w281
              shift-left: w283 -> [w374]
              shift-right: [w341] -> _
              shift-left: 0.0 -> [w339]
              stop <- w421 stop-if-true
              w342 = 4 ("minimum value")
              # "Only update O2 at top of motor cycle"
              # "Ambient condition outputs"
              # "Replace Hall Sensor voltage with motor speed"
              # "Exit Conditions and front panel updates"
              # "Test Loop"
              n177 = local read "Motor Control"() -> (w367:bool)
              n178 = local read "Total Test Time"() -> (w419:i32)
              n179 = call "Elapsed Time"("Time Target (s)"=w419, "Auto Reset"=TRUE ("Reset")) -> ("Elapsed Time (s)"=w365:dbl, "Time has Elapsed"=w420:bool)  [unwired: 10 in, 6 out]
              n180 = local read "Is PAT Test?"() -> (w409:bool)
              n181 = call-poly <vilib>:"DAQmx Read.vi"("task/channels in"=w415, "error in"=w414) -> ("task out"=w412:refnum<k21>, "data"=w386:dbl[], "error out"=w413:errorcluster)  [unwired: 11 in]
              n182 = Array Size(array=w386) -> (size(s)=w387:i32)
              n183 = call-poly <vilib>:"DAQmx Read.vi"("task/channels in"=w393, "error in"=w392) -> ("task out"=w395:refnum<k21>, "data"=w369:dbl[], "error out"=w394:errorcluster)  [unwired: 11 in]
              n184 = Delete From Array(array=w369, index=3 ("dimension size")) -> (deleted portion=w336:dbl, array with subset deleted=w351:dbl[])  [unwired: 1 in]
              n185 = case shown="True" w367 {
                tunnel: w374 -> [w511 w519]
                tunnel: [w511 w518] -> w373
                tunnel: [w510 w517] -> w372
                tunnel: [0.0 ("element") w516] -> w371
                tunnel: w370 -> [w510 w515]
                tunnel: w336 -> [_ w513]
                frame False {
                }
                frame True {
                  # "Motor Control"
                  n186 = call "Elapsed Time2"() -> ("Elapsed Time (s)"=w514:dbl)  [unwired: 12 in, 7 out]
                  n187 = Less?(x=w513, y=2.5) -> (x < y?=w521:bool)
                  n188 = Greater?(x=w514, y=5.0) -> (0:w526:bool)
                  n189 = case shown="False" w521 {
                    tunnel: [w533 w546] -> w518
                    tunnel: w519 -> [w532 w546]
                    tunnel: w515 -> [w531 w545]
                    tunnel: [w530 w545] -> w517
                    tunnel: w526 -> [w528 _]
                    tunnel: w514 -> [w527 _]
                    frame False {
                      n190 = local read "Hit Recorded"() -> (w529:bool)
                      n191 = case shown="True" w529 {
                        tunnel: [w535 w541] -> w533
                        tunnel: w532 -> [w538 w541]
                        tunnel: w531 -> [_ w540]
                        tunnel: [w536 w540] -> w530
                        tunnel: w528 -> [_ w539]
                        tunnel: w527 -> [w535 _]
                        frame False {
                          n192 = Subtract(x=w535, y=w538) -> (x-y=w537:dbl)
                          n193 = local read "Corrected Voltage"() -> (w536:dbl)
                          n194 = local write "Rotation Time"(w537) -> ()
                          n195 = local write "Reference Voltage"(w536) -> ()
                          n196 = local write "Hit Recorded"(TRUE ("Boolean")) -> ()
                        }
                        frame True {
                          n197 = case shown="True" w539 {
                            frame False {
                            }
                            frame True {
                              n198 = local read "Reference Voltage"() -> (w543:dbl)
                              n199 = local read "Error Ratio"() -> (w542:dbl)
                              n200 = Multiply(x=w542, y=w543) -> (x*y=w544:dbl)
                              n201 = local write "Corrected Voltage"(w544) -> ()
                            }
                          }
                        }
                      }
                    }
                    frame True {
                      n202 = local write "Hit Recorded"(FALSE ("Counted")) -> ()
                    }
                  }
                  n203 = local read "Target Rotation Time"() -> (w523:dbl)
                  n204 = local read "Rotation Time"() -> (w522:dbl)
                  n205 = local read "Reference Voltage"() -> (w512:dbl)
                  n206 = Divide(x=w522, y=w523) -> (x/y=w524:dbl)
                  n207 = local write "Error Ratio"(w524) -> ()
                  n208 = call "Motor Safety Limits.vi"("Reference Voltage in"=w512, "Boolean"=w526) -> ("Reference Voltage out"=w516:dbl)  [unwired: 9 in]
                }
              }
              n209 = case shown="True" w409 {
                tunnel: w420 -> [_ w548]
                frame False {
                }
                frame True {
                  n210 = case shown="True" w548 {
                    frame False {
                    }
                    frame True {
                      n211 = local read "Current Test"() -> (w551:string)
                      n212 = local read "Test Status:"() -> (w549:string)
                      n213 = Concatenate Strings(w549, w551, " complete", "\r\n") -> (w550:string)
                      n214 = local write "Test Status:"(w550) -> ()
                    }
                  }
                }
              }
              n215 = Array Size(array=w351) -> (size(s)=w350:i32)
              n216 = local read "Rotation Time"() -> (w349:dbl)
              n217 = local read "Test Buffer Duration"() -> (w366:i32)
              n218 = local read "Stop Custom Test"() -> (w417:bool)
              n219 = local read "Stop PAT Test"() -> (w416:bool)
              n220 = Insert Into Array(array=w351, index=w350, new element=w349) -> (w348:dbl[])
              n221 = Insert Into Array(array=w386, index=w387, new element=w348) -> (w381:dbl[])
              n222 = Index Array(array=w381) -> (element #1=w404:dbl, element #2=w403:dbl, element #3=w401:dbl, element #4=w400:dbl, element #5=w402:dbl, element #6=w399:dbl, element #7=w398:dbl, element #8=w375:dbl, element #9=w347:dbl)  [unwired: 9 in]
              n223 = Build Array(w404, w403, w402, w398, w375, w347) -> (w397:dbl[])
              n224 = Build Array(w401, w400, w399) -> (w396:dbl[])
              n225 = Or(x=w417, y=w416) -> (x .or. y?=w418:bool)
              n226 = Subtract(x=w365, y=w366) -> (x-y=w363:dbl)
              n227 = Less Or Equal?(x=w366, y=w365) -> (x <= y?=w364:bool)
              n228 = case shown="True" w364 {
                tunnel: w411 -> [w428 w433]
                tunnel: w410 -> [w427 w432]
                tunnel: w397 -> [_ w431]
                tunnel: [w428 w430] -> w379
                tunnel: [w427 w429] -> w338
                frame False {
                }
                frame True {
                  n229 = call "Data Manager.vi"("Max Av Values In"=w432, "Data Array In"=w433, "Data"=w431) -> ("Max Av Values Out"=w429:dbl[], "Data Array Out"=w430:dbl[][])  [unwired: 5 in]
                }
              }
              n230 = local write "Stop Test"(w418) -> ()
              n231 = Or(x=w420, y=w418) -> (x .or. y?=w421:bool)
              n232 = Insert Into Array(array=w346, index (col)=0, new element=w396) -> (w352:dbl[][])  [unwired: 1 in]
              n233 = local read "Hit Recorded"() -> (w343:bool)
              n234 = Delete From Array(array=w352, index (col)=100) -> (array with subset deleted=w337:dbl[][])  [unwired: 2 in, 1 out]
              n235 = local read "CV1 Voltage"() -> (w362:dbl)
              n236 = local read "CV2 Voltage"() -> (w361:dbl)
              n237 = Index Array(array=w337) -> (element #1=w407:dbl[], element #2=w406:dbl[], element #3=w405:dbl[])  [unwired: 6 in]
              n238 = Replace Array Subset(array=w338, new element=w339, index=w342) -> (w340:dbl[])
              n239 = case shown="True" w364 {
                tunnel: w340 -> [_ w436]
                tunnel: w363 -> [_ w435]
                frame False {
                }
                frame True {
                  n240 = local read "Test Duration"() -> (w440:i32)
                  n241 = local read "Test Underway"() -> (w443:i32)
                  n242 = local read "In Progress"() -> (w434:bool)
                  n243 = Divide(x=w435, y=w440) -> (x/y=w441:dbl)
                  n244 = Multiply(x=w441, y=100) -> (x*y=w438:dbl)
                  n245 = case shown="False" w434 {
                    frame False {
                      # "Displays 'In Progress'"
                      n246 = local read "Current Test"() -> (w448:string)
                      n247 = local read "Test Status:"() -> (w450:string)
                      n248 = local write "In Progress"(TRUE ("Boolean 2")) -> ()
                      n249 = Concatenate Strings(w450, w448, " in progress...", "\r\n") -> (w449:string)
                      n250 = local write "Test Status:"(w449) -> ()
                      n251 = property on="Test Status:" class="Str"("Text.Scroll Position"=999) -> ()  [unwired: 2 in, 2 out]
                    }
                    frame True {
                    }
                  }
                  n252 = local read "PAT Test Readings"() -> (w442:T1)
                  n253 = case "Test Results" shown="0, Default" w443 {
                    tunnel: w435 -> [_ w471 w478 w485 w492 w499 w506]
                    tunnel: w442 -> [w465 w472 w479 w487 w494 w501 w507]
                    tunnel: w438 -> [_ w470 w477 w484 w491 w498 w505]
                    tunnel: [w465 w473 w480 w486 w493 w500 w508] -> w437
                    tunnel: w436 -> [w464 w468 w475 w482 w488 w496 w502]
                    frame 0, Default {
                      # "Manual Control Test Parameters"
                      n254 = Index Array(array=w464) -> (element #1=w458:dbl, element #2=w457:dbl, element #3=w462:dbl, element #4=w461:dbl, element #5=w460:dbl, element #6=w456:dbl)  [unwired: 6 in]
                      n255 = call "Actuator Output Calculations.vi"("Interval"=w456, "CV1 Voltage"=w457, "CV2 Voltage"=w458) -> ("Motor Speed"=w454:dbl, "CV1 Flow Rate"=w455:dbl, "CV2 Flow Rate"=w459:dbl)  [unwired: 6 in]
                      n256 = call "P1, P2, O2 Calculations.vi"("O2 Voltage"=w460, "P2 Voltage"=w461, "P1 Voltage"=w462) -> ("O2"=w451:dbl, "P2 Pressure"=w453:dbl, "P1 Pressure"=w452:dbl)  [unwired: 6 in]
                      n257 = local read "MC Instrumentation"() -> (w463:T4)
                      n258 = Bundle By Name(cluster=w463, "CV2 Flow Rate:"=w459, "CV1 Flow Rate:"=w455, "Motor Speed:"=w454, "P1 Pressure:"=w452, "P2 Pressure:"=w453, "O2 Concentration:"=w451) -> (w466:T4)
                      n259 = local write "MC Instrumentation"(w466) -> ()
                    }
                    frame 1 {
                      # "Inhalation 30LPM Test Parameters"
                      n260 = Index Array(array=w468, index=4 ("minimum value")) -> (element=w469:dbl)
                      n261 = Bundle By Name(cluster=w472, "In30 T"=w471, "In30 S"=w470, "In30 M"=w469) -> (w473:T1)
                    }
                    frame 2 {
                      # "Inhalation 70LPM Test Parameters"
                      n262 = Index Array(array=w475, index=4 ("minimum value")) -> (element=w474:dbl)
                      n263 = Bundle By Name(cluster=w479, "In70 T"=w478, "In70 S"=w477, "In70 M"=w474) -> (w480:T1)
                    }
                    frame 3 {
                      # "Exhalation 30LPM Test Parameters"
                      n264 = Index Array(array=w482, index=4 ("minimum value")) -> (element=w481:dbl)
                      n265 = Bundle By Name(cluster=w487, "Ex30 T"=w485, "Ex30 S"=w484, "Ex30 M"=w481) -> (w486:T1)
                    }
                    frame 4 {
                      # "Exhalation 70LPM Test Parameters"
                      n266 = Index Array(array=w488, index=4 ("minimum value")) -> (element=w489:dbl)
                      n267 = Bundle By Name(cluster=w494, "Ex70 T"=w492, "Ex70 S"=w491, "Ex70 M"=w489) -> (w493:T1)
                    }
                    frame 5 {
                      # "Breathing 15kft Test Output"
                      n268 = Index Array(array=w496, index=4 ("minimum value")) -> (element=w495:dbl)
                      n269 = Bundle By Name(cluster=w501, "B15 T"=w499, "B15 S"=w498, "B15 M"=w495) -> (w500:T1)
                    }
                    frame 6 {
                      # "Breathing 40kft Test Output"
                      n270 = Index Array(array=w502, index=4 ("minimum value")) -> (element=w503:dbl)
                      n271 = Bundle By Name(cluster=w507, "B40 T"=w506, "B40 S"=w505, "B40 M"=w503) -> (w508:T1)
                    }
                  }
                  n272 = local write "PAT Test Readings"(w437) -> ()
                }
              }
              n273 = call-poly <vilib>:"Mean.vi"("X"=w407) -> ("mean"=w354:dbl)  [unwired: 1 out]
              n274 = call-poly <vilib>:"Mean.vi"("X"=w406) -> ("mean"=w355:dbl)  [unwired: 1 out]
              n275 = call-poly <vilib>:"Mean.vi"("X"=w405) -> ("mean"=w356:dbl)  [unwired: 1 out]
              n276 = case shown="True" w343 {
                tunnel: w338 -> [_ w426]
                tunnel: [w423 w425] -> w341
                tunnel: w339 -> [w423 _]
                tunnel: w342 -> [_ w424]
                frame False {
                }
                frame True {
                  n277 = Index Array(array=w426, index=w424) -> (element=w425:dbl)
                }
              }
              n278 = Build Array(w362, w361) -> (w345:dbl[])
              n279 = call "Ambient Sensor Calculations.vi"("PA Voltage"=w356, "RHA Voltage"=w355, "TA Voltage"=w354) -> ("PA"=w357:dbl, "RHA"=w353:dbl, "TA"=w358:dbl)  [unwired: 6 in]
              n280 = call "CV Voltage Limits.vi"("CV Voltage In"=w345) -> ("CV Voltage Out"=w344:dbl[])  [unwired: 10 in]
              n281 = local read "MC Instrumentation"() -> (w360:T4)
              n282 = Bundle By Name(cluster=w360, "Ambient Temp.:"=w358, "Ambient Humidity:"=w353, "Ambient Pressure:"=w357) -> (w359:T4)
              n283 = local write "MC Instrumentation"(w359) -> ()
              n284 = Delete From Array(array=w379, index (col)=5) -> (array with subset deleted=w378:dbl[][])  [unwired: 2 in, 1 out]
              n285 = call-poly <vilib>:"DAQmx Write.vi"("task/channels in"=w391, "data"=w344, "error in"=w390) -> ("task out"=w389:refnum<k21>, "error out"=w388:errorcluster)  [unwired: 10 in, 1 out]
              n286 = call-poly <vilib>:"DAQmx Write.vi"("task/channels in"=w382, "data"=w371, "error in"=w383) -> ("task out"=w384:refnum<k21>, "error out"=w385:errorcluster)  [unwired: 10 in, 1 out]
              n287 = Delete From Array(array=w338) -> (array with subset deleted=w377:dbl[])  [unwired: 2 in, 1 out]
            }
            n288 = local write "Test Underway"(w319) -> ()
            n289 = case "Test Params" shown="0, Default" w319 {
              tunnel: [w569 15 15 15 15 15 15] -> w277
              tunnel: [w570 "Inhalation 30LPM" "Inhalation 70LPM" "Exhalation 30LPM" "Exhalation 70LPM" "Breathing 15kft" "Breathing 40kft"] -> w318
              tunnel: [w570 w592 w613 w635 w658 w679 w701] -> w317
              tunnel: [w568 FALSE FALSE FALSE FALSE TRUE TRUE] -> w316
              tunnel: [w567 FALSE ("element") FALSE ("element") FALSE ("element") FALSE ("element") TRUE ("element") TRUE ("element")] -> w315
              tunnel: [w566 FALSE ("element") FALSE ("element") FALSE ("element") FALSE ("element") TRUE ("element") TRUE ("element")] -> w314
              tunnel: [w565 TRUE ("element") TRUE ("element") TRUE ("element") TRUE ("element") TRUE ("element") TRUE ("element")] -> w313
              tunnel: [w558 FALSE ("element") FALSE ("element") FALSE ("element") FALSE ("element") TRUE ("element") TRUE ("element")] -> w312
              tunnel: [w561 TRUE ("element") TRUE ("element") FALSE ("element") FALSE ("element") FALSE ("element") FALSE ("element")] -> w311
              tunnel: [w562 TRUE ("element") TRUE ("element") FALSE ("element") FALSE ("element") FALSE ("element") FALSE ("element")] -> w310
              tunnel: [w560 FALSE ("element") FALSE ("element") TRUE ("element") TRUE ("element") FALSE ("element") FALSE ("element")] -> w304
              tunnel: [w563 FALSE ("element") FALSE ("element") TRUE ("element") TRUE ("element") FALSE ("element") FALSE ("element")] -> w309
              tunnel: [w559 FALSE ("element") FALSE ("element") FALSE ("element") FALSE ("element") TRUE ("element") TRUE ("element")] -> w279
              tunnel: [w564 TRUE ("element") TRUE ("element") TRUE ("element") TRUE ("element") FALSE ("element") FALSE ("element")] -> w308
              tunnel: [w557 FALSE ("element") FALSE ("element") FALSE ("element") FALSE ("element") TRUE ("element") TRUE ("element")] -> w307
              tunnel: [w556 30.0 70.0 30.0 70.0 0.0 0.0] -> w271
              tunnel: [w554 0.0 0.0 0.0 0.0 1.0 5.0] -> w270
              tunnel: [w555 0.0 0.0 0.0 0.0 0.357142857 0.357142857] -> w269
              frame 0, Default {
                w570 = ""
                # "Manual Control Test Parameters"
                n290 = local read "MC Instrumentation"() -> (w571:T4)
                n291 = Unbundle By Name(w571) -> ("SV1"=w568:bool, "SV2"=w567:bool, "SV3"=w566:bool, "SV4"=w565:bool, "SV5"=w558:bool, "SV6"=w561:bool, "SV7"=w562:bool, "SV8"=w560:bool, "SV9"=w563:bool, "M1"=w559:bool, "MP1"=w564:bool, "MP2"=w557:bool, "Motor Speed:"=w555:dbl, "CV1 Flow Rate:"=w554:dbl, "CV2 Flow Rate:"=w556:dbl)
                n292 = local read "MC Fields"() -> (w572:T3)
                n293 = Unbundle By Name(w572) -> ("MC Test Length"=w573:enum32{"Run Continuously", "Run for:"})
                n294 = case shown="\"Run Continuously\", Default" w573 {
                  tunnel: [2100000000 w575] -> w569
                  frame "Run Continuously", Default {
                  }
                  frame "Run for:" {
                    n295 = local read "MC Fields"() -> (w576:T3)
                    n296 = Unbundle By Name(w576) -> ("Test Duration"=w575:i64)
                  }
                }
              }
              frame 1 {
                # "Inhalation 30LPM Test Parameters"
                n297 = property on="Test Status:" class="Str"("Text.Scroll Position"=999) -> ()  [unwired: 2 in, 2 out]
                n298 = Concatenate Strings("Inhalation 30LPM initialising...", "\r\n") -> (w592:string)
              }
              frame 2 {
                # "Inhalation 70LPM Test Parameters"
                n299 = property on="Test Status:" class="Str"("Text.Scroll Position"=999) -> ()  [unwired: 2 in, 2 out]
                n300 = local read "Test Status:"() -> (w616:string)
                n301 = Concatenate Strings(w616, "Inhalation 70LPM test initialising...", "\r\n") -> (w613:string)
              }
              frame 3 {
                # "Exhalation 30LPM Test Parameters"
                n302 = property on="Test Status:" class="Str"("Text.Scroll Position"=999) -> ()  [unwired: 2 in, 2 out]
                n303 = local read "Test Status:"() -> (w638:string)
                n304 = Concatenate Strings(w638, "Exhalation 30LPM initialising...", "\r\n") -> (w635:string)
              }
              frame 4 {
                # "Exhalation 70LPM Test Parameters"
                n305 = property on="Test Status:" class="Str"("Text.Scroll Position"=999) -> ()  [unwired: 2 in, 2 out]
                n306 = local read "Test Status:"() -> (w660:string)
                n307 = Concatenate Strings(w660, "Exhalation 70LPM initialising...", "\r\n") -> (w658:string)
              }
              frame 5 {
                # "Breathing 15kft Test Parameters"
                n308 = property on="Test Status:" class="Str"("Text.Scroll Position"=999) -> ()  [unwired: 2 in, 2 out]
                n309 = local read "Test Status:"() -> (w682:string)
                n310 = Concatenate Strings(w682, "Breathing 15kft test initialising...", "\r\n") -> (w679:string)
              }
              frame 6 {
                # "Breathing 40kft Test Parameters"
                n311 = property on="Test Status:" class="Str"("Text.Scroll Position"=999) -> ()  [unwired: 2 in, 2 out]
                n312 = local read "Test Status:"() -> (w704:string)
                n313 = Concatenate Strings(w704, "Breathing 40kft test initialising...", "\r\n") -> (w701:string)
              }
            }
            n314 = local read "Test Buffer Duration"() -> (w278:i32)
            n315 = Add(x=w278, y=w277) -> (x+y=w276:i64)
            n316 = Build Array(w316, w315, w314, w313, w312, w311, w310, w304, w309, w279, w308, w307) -> (w306:bool[])
            n317 = Array Size(array=w306) -> (size(s)=w305:i32)
            n318 = call "Actuator Calculations.vi"("CV2 Flow Rate:"=w271, "CV1 Flow Rate:"=w270, "Motor Speed:"=w269) -> ("CV2 Voltage"=w273:dbl, "CV1 Voltage"=w272:dbl, "Interval"=w274:dbl)  [unwired: 6 in]
            n319 = for {
              N: w305 -> [_]
              tunnel: w306 -> [w334] mode=indexing
              tunnel: [w331] -> w303
              tunnel: [w330] -> w302
              tunnel: w301 -> [w327]
              tunnel: w300 -> [w326]
              i -> [w335]
              # "Relay Control"
              n320 = call "Relay Command Generator.vi"("Relay"=w335, "On/Off"=w334) -> ("Generated Command"=w333:string)  [unwired: 8 in]
              n321 = Concatenate Strings(w333, "\n" ("string")) -> (w329:string)
              n322 = VISA Write(VISA resource name=w327, write buffer=w329, error in (no error)=w326) -> (VISA resource name out=w330:refnum<visa-resource-name>, error out=w331:errorcluster)  [unwired: 1 out]
              n323 = Wait (ms)(milliseconds to wait=u32 20) -> ()  [unwired: 1 out]
            }
            n324 = local write "Total Test Time"(w276) -> ()
            n325 = local write "Test Duration"(w277) -> ()
            n326 = local write "Test Status:"(w317) -> ()
            n327 = local write "Current Test"(w318) -> ()
            n328 = local write "Motor Control"(w279) -> ()
            n329 = local write "Target Rotation Time"(w274) -> ()
            n330 = local write "CV1 Voltage"(w272) -> ()
            n331 = local write "CV2 Voltage"(w273) -> ()
            n332 = local write "In Progress"(FALSE ("In Progress")) -> ()
          }
          frame True {
          }
        }
      }
      n333 = for {
        N: 10 -> [_]
        tunnel: w210 -> [w240]
        tunnel: w209 -> [w239]
        tunnel: [w238] -> w208
        tunnel: [w237] -> w207
        n334 = Concatenate Strings("\":FE0F00000010020000E1\"" ("write buffer"), "\n" ("string")) -> (w236:string)
        n335 = VISA Write(VISA resource name=w239, write buffer=w236, error in (no error)=w240) -> (VISA resource name out=w237:refnum<visa-resource-name>, error out=w238:errorcluster)  [unwired: 1 out]
      }
      n336 = local write "Reference Voltage"(w146) -> ()
      n337 = call <vilib>:"DAQmx Stop Task.vi"("task/channels in"=w229, "error in"=w228) -> ("task out"=w227:refnum<k21>, "error out"=w226:errorcluster)  [unwired: 12 in]
      n338 = call <vilib>:"DAQmx Stop Task.vi"("task/channels in"=w204, "error in"=w203) -> ("task out"=w206:refnum<k21>, "error out"=w205:errorcluster)  [unwired: 12 in]
      n339 = call <vilib>:"DAQmx Stop Task.vi"("task/channels in"=w183, "error in"=w182) -> ("task out"=w193:refnum<k21>, "error out"=w194:errorcluster)  [unwired: 12 in]
      n340 = call <vilib>:"DAQmx Stop Task.vi"("task/channels in"=w166, "error in"=w167) -> ("task out"=w159:refnum<k21>, "error out"=w158:errorcluster)  [unwired: 12 in]
      n341 = call <vilib>:"DAQmx Clear Task.vi"("task in"=w227, "error in"=w226) -> ("error out"=w198:errorcluster)  [unwired: 13 in]
      n342 = call <vilib>:"DAQmx Clear Task.vi"("task in"=w206, "error in"=w205) -> ("error out"=w200:errorcluster)  [unwired: 13 in]
      n343 = call <vilib>:"DAQmx Clear Task.vi"("task in"=w193, "error in"=w194) -> ("error out"=w195:errorcluster)  [unwired: 13 in]
      n344 = call <vilib>:"DAQmx Clear Task.vi"("task in"=w159, "error in"=w158) -> ("error out"=w157:errorcluster)  [unwired: 13 in]
      n345 = call <vilib>:"Simple Error Handler.vi"("type of dialog (OK msg:1)"=w197, "error in (no error)"=w198) -> ()  [unwired: 3 in, 5 out]
      n346 = call <vilib>:"Simple Error Handler.vi"("type of dialog (OK msg:1)"=w199, "error in (no error)"=w200) -> ()  [unwired: 3 in, 5 out]
      n347 = call <vilib>:"Simple Error Handler.vi"("type of dialog (OK msg:1)"=w196, "error in (no error)"=w195) -> ()  [unwired: 3 in, 5 out]
      n348 = call <vilib>:"Simple Error Handler.vi"("type of dialog (OK msg:1)"=w156, "error in (no error)"=w157) -> ()  [unwired: 3 in, 5 out]
      n349 = VISA Close(VISA resource name=w207, error in (no error)=w208) -> (error out=w212:errorcluster)
      n350 = call <vilib>:"Simple Error Handler.vi"("error in (no error)"=w212) -> ()  [unwired: 1 in, 8 out]
    }
  }
  n351 = case "Test Exit" shown="True" w25 {
    tunnel: [FALSE w729] -> w20
    frame False {
    }
    frame True {
      w728 = FALSE
      n352 = local read "Stop Test"() -> (w731:bool)
      n353 = property on="Test Status:" class="Str"("Text.Scroll Position"=999) -> ()  [unwired: 2 in, 2 out]
      n354 = case "Exit Type" shown="True" w731 {
        frame False {
          n355 = local read "Test Status:"() -> (w732:string)
          n356 = Concatenate Strings(w732, "All tests complete") -> (w733:string)
          n357 = local write "Test Status:"(w733) -> ()
        }
        frame True {
          n358 = local read "Test Status:"() -> (w736:string)
          n359 = Concatenate Strings(w736, "Testing Cancelled") -> (w737:string)
          n360 = local write "Test Status:"(w737) -> ()
        }
      }
      n361 = local read "Is PAT Test?"() -> (w729:bool)
      n362 = local write "Start Custom Test"(w728) -> ()
      n363 = local write "Start PAT Test"(w728) -> ()
      n364 = local write "Test Begin"(w728) -> ()
      n365 = local write "Motor Control"(w728) -> ()
    }
  }
  n366 = case "Save Report" shown="True" w20 {
    frame False {
    }
    frame True {
      # "Save report"
      # "Report Title"
      # "Collect data headings for report"
      # "Collect data for report"
      n367 = local read "PAT Test Readings"() -> (w764:T1)
      n368 = local read "PAT Test Settings"() -> (w765:T2)
      n369 = property on="String" class="Str"() -> ("Value"=w763:string)  [unwired: 2 in, 2 out]
      n370 = property on="String 2" class="Str"() -> ("Value"=w739:string)  [unwired: 2 in, 2 out]
      n371 = property on="String 3" class="Str"() -> ("Value"=w762:string)  [unwired: 2 in, 2 out]
      n372 = property on="String 4" class="Str"() -> ("Value"=w761:string)  [unwired: 2 in, 2 out]
      n373 = property on="String 5" class="Str"() -> ("Value"=w760:string)  [unwired: 2 in, 2 out]
      n374 = property on="String 6" class="Str"() -> ("Value"=w738:string)  [unwired: 2 in, 2 out]
      n375 = property on="Test Date:" class="Str"() -> ("Label.Text"=w778:string)  [unwired: 2 in, 2 out]
      n376 = property on="Test Time:" class="Str"() -> ("Label.Text"=w779:string)  [unwired: 2 in, 2 out]
      n377 = property on="Pull Test Date:" class="Str"() -> ("Label.Text"=w780:string)  [unwired: 2 in, 2 out]
      n378 = property on="Operator:" class="Str"() -> ("Label.Text"=w781:string)  [unwired: 2 in, 2 out]
      n379 = property on="Production Order No.:" class="Str"() -> ("Label.Text"=w782:string)  [unwired: 2 in, 2 out]
      n380 = property on="Production Lot:" class="Str"() -> ("Label.Text"=w783:string)  [unwired: 2 in, 2 out]
      n381 = property on="No. Masks in Lot:" class="Str"() -> ("Label.Text"=w784:string)  [unwired: 2 in, 2 out]
      n382 = property on="Facepiece Leakage" class="DigNum (strict)"() -> ("Label.Text"=w785:string)  [unwired: 2 in, 2 out]
      n383 = property on="Comments:" class="Str"() -> ("Label.Text"=w786:string)  [unwired: 2 in, 2 out]
      n384 = Unbundle By Name(w765) -> ("Test Date:"=w742:string, "Test Time:"=w744:string, "Pull Test Date:"=w771:string, "Operator:"=w772:string, "Production Order No.:"=w770:string, "No. Masks in Lot:"=w773:string, "Production Lot:"=w774:string, "Comments:"=w775:string, "Facepiece Leakage"=w755:dbl)
      n385 = Unbundle By Name(w764) -> ("In30 M"=w754:dbl, "In70 M"=w753:dbl, "Ex30 M"=w752:dbl, "Ex70 M"=w751:dbl, "B15 M"=w741:dbl, "B40 M"=w750:dbl)
      n386 = property on="Ambient Humidity:" class="DigNum (strict)"() -> ("Value"=w740:dbl)  [unwired: 2 in, 2 out]
      n387 = property on="Ambient Pressure:" class="DigNum (strict)"() -> ("Value"=w749:dbl)  [unwired: 2 in, 2 out]
      n388 = property on="Ambient Temp.:" class="DigNum (strict)"() -> ("Value"=w748:dbl)  [unwired: 2 in, 2 out]
      n389 = property on="Ambient Humidity:" class="DigNum (strict)"() -> ("Label.Text"=w759:string)  [unwired: 2 in, 2 out]
      n390 = property on="Ambient Pressure:" class="DigNum (strict)"() -> ("Label.Text"=w758:string)  [unwired: 2 in, 2 out]
      n391 = property on="Ambient Temp.:" class="DigNum (strict)"() -> ("Label.Text"=w757:string)  [unwired: 2 in, 2 out]
      n392 = Build Array(w778, w779, w780, w781, w782, w783, w784, w785, w786, w763, w739, w762, w761, w760, w738, w759, w758, w757) -> (w767:string[])
      n393 = Build Array(w755, w754, w753, w752, w751, w741, w750, w740, w749, w748) -> (w756:dbl[])
      n394 = Number To Fractional String(number=w756, precision (6)=3) -> (F-format string=w746:string[])  [unwired: 2 in]
      n395 = Build Array(w742, w744, w771, w772, w770, w773, w774, w775) -> (w747:string[])
      n396 = Insert Into Array(array=w747, new element=w746) -> (w743:string[])  [unwired: 1 in]
      n397 = local read "Results File Location:"() -> (w768:path)
      n398 = Concatenate Strings(w770, " Testing - ", w742) -> (w766:string)
      n399 = call "Save Report SubVI.vi"("File Name"=w766, "error in (no error)"="error in (no error)", "Value Names"=w767, "Values"=w743, "Results File Location:"=w768) -> ("error out"=→"error out":errorcluster)  [unwired: 6 in]
    }
  }
